vi "TestUsbSerialPort.vi"(7 "DTR Delay":dbl=0.25, 8 "Error In":errorcluster, 11 "Serial Port To Test":refnum<visa-resource-name>) -> (0 "Error Out":errorcluster, 3 "Output Serial Port":refnum<visa-resource-name>)   [LabVIEW 2010]
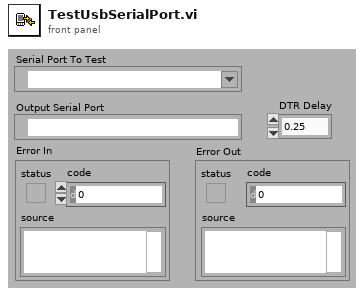
[diagram p1: front panel]
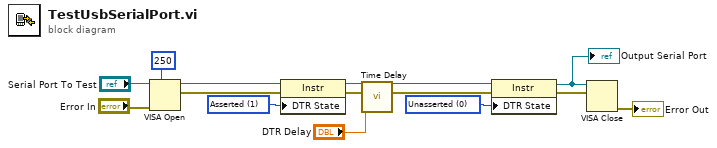
[diagram p0: block diagram]
diagram:
  w4 = i16 0 items=["Unknown"=-1, "Unasserted"=0, "Asserted"=1] ("Serial Settings:Modem Line Settings:Line DTR State")
  w12 = i16 1 items=["Unknown"=-1, "Unasserted"=0, "Asserted"=1] ("Serial Settings:Modem Line Settings:Line DTR State")
  n1 = VISA Open(timeout (0)=u32 250 ("VISA Open timeout (0)"), error in (no error)="Error In", VISA resource name="Serial Port To Test") -> (VISA resource name=w10:refnum<visa-resource-name>, error out=w11:errorcluster)  [unwired: 2 in]
  n2 = property class="Instr"(reference=w10, error in=w11, "DTR State"=w12) -> (reference out=w6:refnum<visa-resource-name>, error out=w7:errorcluster)
  n3 = call "Time Delay"("error in (no error)"=w7, "Delay Time (s)"="DTR Delay") -> ("error out"=w5:errorcluster)  [unwired: 9 in]
  n4 = property class="Instr"(reference=w6, error in=w5, "DTR State"=w4) -> (reference out=w3:refnum<visa-resource-name>, error out=w2:errorcluster)
  "Output Serial Port" <- w3
  n5 = VISA Close(VISA resource name=w3, error in (no error)=w2) -> (error out=→"Error Out":errorcluster)
